vi "Scale Camera Parameters to New Size.vi"(1 "New Size":T2, 2 "Current Size":T2, 3 "Camera Matrix":T1) -> (0 "Scaled Camera Matrix":T1)   [LabVIEW 2020, in "ar.lvlib"]
doc: "Scale a Camera Matrix to a new size. This can be used to obtain a reasonable approximation of a Camera Matrix computed for one image size at an alternative image size."
uses:
  ar.lvlib
  common/Image Size (Integer).ctl
  common/Camera Matrix.ctl
  common/common.lvlib
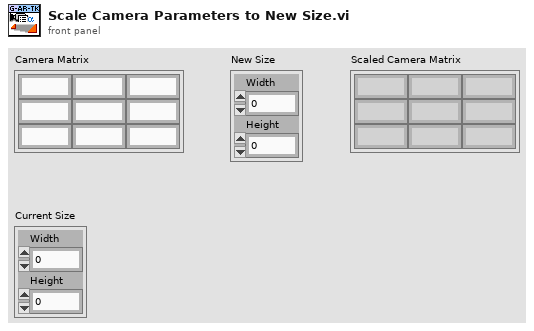
[diagram p1: front panel]
types:
  T1 = typedef "common.lvlib/Camera Matrix.ctl" = cluster{"m 0,0":dbl, "m 0,1":dbl, "m 0,2":dbl, "m 1,0":dbl, "m 1,1":dbl, "m 1,2":dbl, "m 2,0":dbl, "m 2,1":dbl, "m 2,2":dbl}
  T2 = typedef "common.lvlib/Image Size (Integer).ctl" = cluster{"Width":u16, "Height":u16}
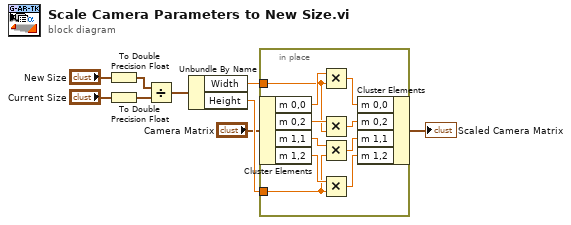
[diagram p0: block diagram]
diagram:
  n1 = To Double Precision Float(number="New Size") -> (double precision float=w9:cluster{"Width":dbl, "Height":dbl})
  n2 = To Double Precision Float(number="Current Size") -> (double precision float=w8:cluster{"Width":dbl, "Height":dbl})
  n3 = Divide(x=w9, y=w8) -> (x/y=w7:cluster{"Width":dbl, "Height":dbl})
  n4 = Unbundle By Name(w7) -> ("Width"=w6:dbl, "Height"=w5:dbl)
  n5 = in-place {
    in-place-border: w6 -> [w17]
    in-place-border: w5 -> [w10]
    n6 = in-place-cluster #1("Camera Matrix") -> ("m 0,0"=w19:dbl, "m 0,2"=w18:dbl, "m 1,1"=w14:dbl, "m 1,2"=w12:dbl)
    n7 = Multiply(x=w19, y=w17) -> (x*y=w15:dbl)
    n8 = Multiply(x=w18, y=w17) -> (x*y=w16:dbl)
    n9 = Multiply(x=w14, y=w10) -> (x*y=w13:dbl)
    n10 = Multiply(x=w12, y=w10) -> (x*y=w11:dbl)
    n11 = in-place-cluster #1("m 0,0"=w15, "m 0,2"=w16, "m 1,1"=w13, "m 1,2"=w11) -> (→"Scaled Camera Matrix":T1)
  }
